vi "LockinDAQ.Configure Sweep 1.vi"(8 "error in (no error)":errorcluster, 11 "LockinDAQ in":refnum<class "LockinDAQ.lvclass">) -> (0 "error out":errorcluster, 3 "LockinDAQ out":refnum<class "LockinDAQ.lvclass">)   [LabVIEW 2016, in "LockinDAQ.lvclass"]
uses:
  LockinDAQ.lvclass
  Typedefs/Function-enum.ctl
  LockinDAQ.lvclass/LockinDAQ.ctl
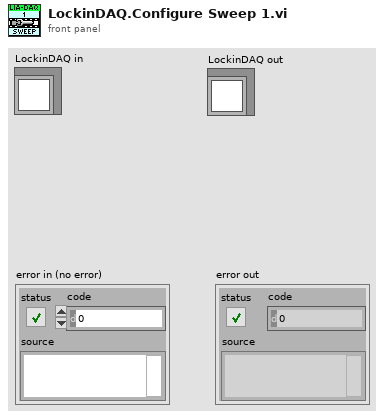
[diagram p1: front panel]
types:
  T1 = typedef "LockinDAQ.lvclass/Function-enum.ctl" = enum16{"Sine", "Triangle", "Square", "Sawtooth"}
  T2 = typedef "LockinDAQ.lvclass/AO-cluster.ctl" = cluster{"AO Amp (V)":T3, "AO DC (V)":T4, "AO f (Hz)":T5, "AO Phase (°)":T6, "Function":T7, "I+":bool[], "Sweeping":bool[]}
  T3 = typedef "LockinDAQ.lvclass/AO_Amp-array.ctl" = dbl[]
  T4 = typedef "LockinDAQ.lvclass/AO_DC-array.ctl" = dbl[]
  T5 = typedef "LockinDAQ.lvclass/AO_f-array.ctl" = dbl[]
  T6 = typedef "LockinDAQ.lvclass/AO_phi-array.ctl" = dbl[]
  T7 = typedef "LockinDAQ.lvclass/Function-array.ctl" = T1[]
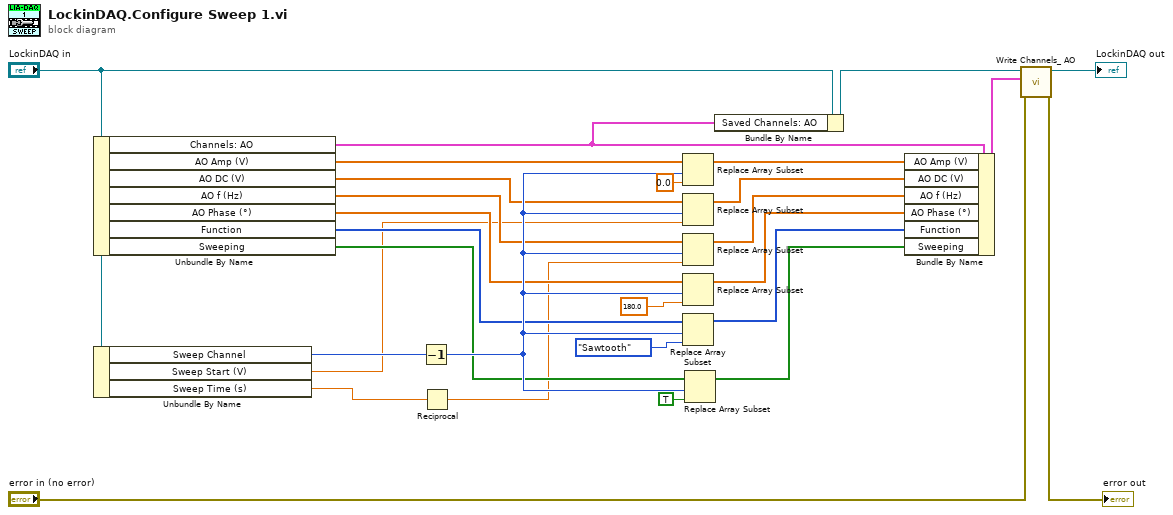
[diagram p0: block diagram]
diagram:
  n1 = Unbundle By Name("LockinDAQ in") -> ("Channels: AO"=w3:T2, "AO Amp (V)"=w20:T3, "AO DC (V)"=w19:T4, "AO f (Hz)"=w18:T5, "AO Phase (°)"=w17:T6, "Function"=w16:T7, "Sweeping"=w15:bool[])
  n2 = Unbundle By Name("LockinDAQ in") -> ("Sweep Channel"=w8:i32, "Sweep Start (V)"=w6:dbl, "Sweep Time (s)"=w2:dbl)
  n3 = Decrement(x=w8) -> (x-1=w21:i32)
  n4 = Reciprocal(x=w2) -> (1/x=w1:dbl)
  n5 = Replace Array Subset(array=w20, new element=0.0 ("new element/subarray"), index=w21) -> (w14:T3)
  n6 = Replace Array Subset(array=w19, new element=w6, index=w21) -> (w13:T4)
  n7 = Replace Array Subset(array=w18, new element=w1, index=w21) -> (w12:T5)
  n8 = Replace Array Subset(array=w17, new element=180.0 ("new element/subarray"), index=w21) -> (w11:T6)
  n9 = Replace Array Subset(array=w16, new element=Function-enum."Sawtooth" ("new element/subarray"), index=w21) -> (w10:T7)
  n10 = Replace Array Subset(array=w15, new element=TRUE ("new element/subarray"), index=w21) -> (w9:bool[])
  n11 = Bundle By Name(cluster="LockinDAQ in", "Saved Channels: AO"=w3) -> (w4:refnum<class "LockinDAQ.lvclass">)
  n12 = Bundle By Name(cluster=w3, "AO Amp (V)"=w14, "AO DC (V)"=w13, "AO f (Hz)"=w12, "AO Phase (°)"=w11, "Function"=w10, "Sweeping"=w9) -> (w25:T2)
  n13 = call "Write Channels_ AO.vi"("error in (no error)"="error in (no error)", "Channels: AO"=w25, "LockinDAQ"=w4) -> ("error out"=→"error out":errorcluster, "LockinDAQ out"=→"LockinDAQ out":refnum<class "LockinDAQ.lvclass">)  [unwired: 7 in]
